vi "218_Test.vi"() -> ()   [LabVIEW 2013]
uses:
  <vilib>/Instr/_visa.llb/VISA Configure Serial Port (Instr).vi
panel:
  out "read buffer":string
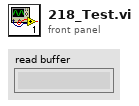
[diagram p1: front panel]
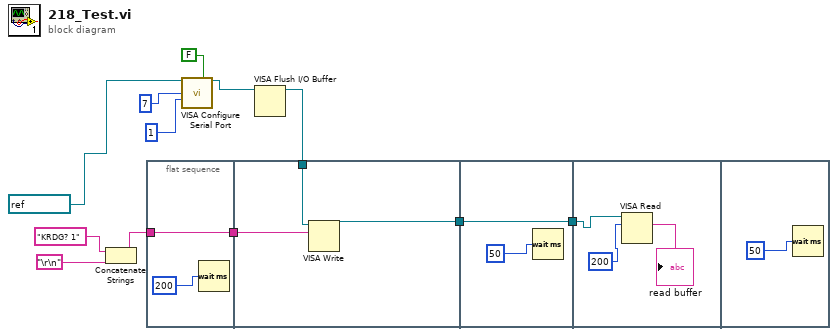
[diagram p0: block diagram]
diagram:
  n1 = Concatenate Strings("KRDG? 1" ("write buffer"), "\r\n") -> (w11:string)
  n2 = flat-sequence {
    tunnel: w11 -> [w14]
    tunnel: [w14] -> w8
    tunnel: [w16] -> w10
    tunnel: w8 -> [w17]
    tunnel: w3 -> [w15]
    tunnel: w10 -> [w18]
    tunnel: [w18] -> w9
    tunnel: w9 -> [w21]
    frame #0 {
      n3 = Wait (ms)(milliseconds to wait=200) -> ()  [unwired: 1 out]
    }
    frame #1 {
      n4 = VISA Write(VISA resource name=w15, write buffer=w17) -> (VISA resource name out=w16:refnum<visa-resource-name>)  [unwired: 1 in, 2 out]
    }
    frame #2 {
      n5 = Wait (ms)(milliseconds to wait=50) -> ()  [unwired: 1 out]
    }
    frame #3 {
      n6 = VISA Read(VISA resource name=w21, byte count=u32 200) -> (read buffer=→"read buffer":string)  [unwired: 1 in, 3 out]
    }
    frame #4 {
      n7 = Wait (ms)(milliseconds to wait=50) -> ()  [unwired: 1 out]
    }
  }
  n8 = call-poly "VISA Configure Serial Port"("VISA resource name"=refnum<visa-resource-name> "COM3", "Enable Termination\nChar (T)"=FALSE, "data bits (8)"=7, "parity (0:none)"=1) -> ("VISA resource name out"=w4:refnum<visa-resource-name>)  [unwired: 10 in, 1 out]
  n9 = VISA Flush I/O Buffer(VISA resource name=w4) -> (VISA resource name out=w3:refnum<visa-resource-name>)  [unwired: 2 in, 1 out]
